vi "Configure IODIR.vi"(8 "error in (no error)":errorcluster, 11 "MCP23017 In":refnum<class "MCP23017.lvclass">) -> (0 "error out":errorcluster, 3 "MCP23017 Out":refnum<class "MCP23017.lvclass">)   [LabVIEW 2020, in "MCP23017.lvclass"]
uses:
  MCP23017.lvclass
  Registers.ctl
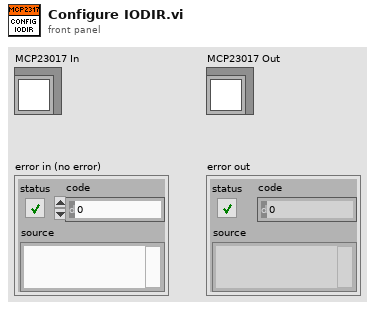
[diagram p1: front panel]
types:
  T1 = typedef "MCP23017.lvclass/Registers.ctl" = u16
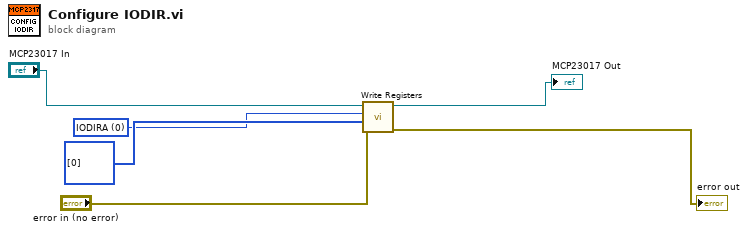
[diagram p0: block diagram]
diagram:
  w1 = T1 0 items=["IODIRA"]
  n1 = call "Write Registers.vi"("error in (no error)"="error in (no error)", "Data"=u8[] [0], "Registers"=w1, "MCP23017 in"="MCP23017 In") -> ("error out"=→"error out":errorcluster, "MCP23017 out"=→"MCP23017 Out":refnum<class "MCP23017.lvclass">)  [unwired: 6 in]
